vi "processString.vi"(8 "error in (no error)":errorcluster, 10 "Message in":string, 11 "SimpleStringMessage in":refnum<class "SimpleStringMessage.lvclass">) -> (0 "error out":errorcluster, 1 "found?":bool, 2 "response":T1, 3 "SimpleStringMessage out":refnum<class "SimpleStringMessage.lvclass">, 4 "isAck?":bool, 5 "Remaining buffer":string)   [LabVIEW 2025, in "SimpleStringMessage.lvclass"]
doc: "Parses and interpretes the input string. If a complete packet from the remote host is found, \"found?\" should return TRUE. In that the case, the response should contain the type and the message data in the variant. \nIf the found message is an acknowledgement to the \"Sent message in\", the isAck? boolean should return TRUE.\nAnything left in the Message in string after the first message has been found should be returned in Remaining buffer"
uses:
  SimpleStringMessage.lvclass
  response.ctl
  driver_status.ctl
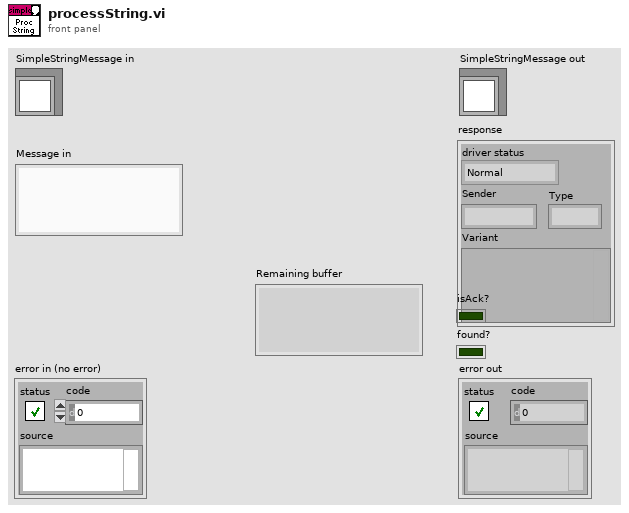
[diagram p1: front panel]
types:
  T1 = typedef "response.ctl" = cluster{"driver status":T2, "Sender":string, "Type":i32, "Variant":variant}
  T2 = typedef "driver_status.ctl" = enum16{"Normal", "Startup", "Connection lost", "Reconnected", "Timeout", "Idle", "Busy"}
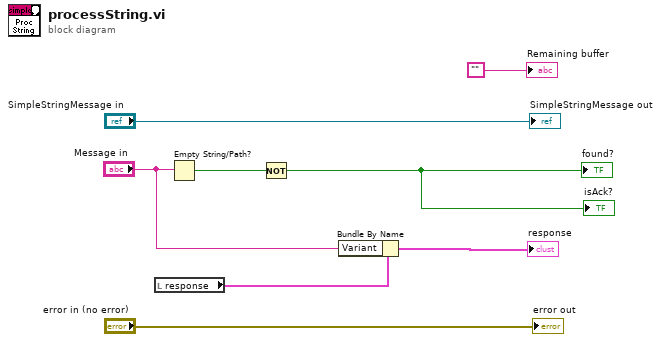
[diagram p0: block diagram]
diagram:
  n1 = local read "response"() -> (w6:T1)
  n2 = Empty String/Path?(string/path="Message in") -> (empty?=w3:bool)
  n3 = Not(x=w3) -> (.not. x?=→"isAck?" →"found?":bool)
  n4 = Bundle By Name(cluster=w6, "Variant"="Message in") -> (→"response":T1)
  "error out" <- "error in (no error)"
  "SimpleStringMessage out" <- "SimpleStringMessage in"
  "Remaining buffer" <- "" ("Empty String Constant")
